vi "MathCad_Easy_NumComplex_Get_Var.vi"(8 "error in (no error)":errorcluster, 9 "Variable  Name":string, 11 "Mathcad Reference":T1) -> (0 "error out":errorcluster, 1 "value":cdb format="%.2f", 3 "Mathcad Reference":T1)   [LabVIEW 2015]
doc: "Sets a Numeric value in Mathcad. You can also use this VI to reset a variable that has already been set once. It is only dependent upon the variable name. The variable won't appear in the Mathcad worksheet, but is defined at the very beginning of the worksheet.\nInputs \n Wrksht Ref--ActiveX Reference to Mathcad Worksheet Class\n Data In--Name and Value of Variable to Set\n Cluster (2 elements)\n Value (Double)\n New Variable Name(String)\nOutputs \n Wrksht Ref--ActiveX Reference to Mathcad Worksheet Class"
uses:
  Mathcad Reference.ctl
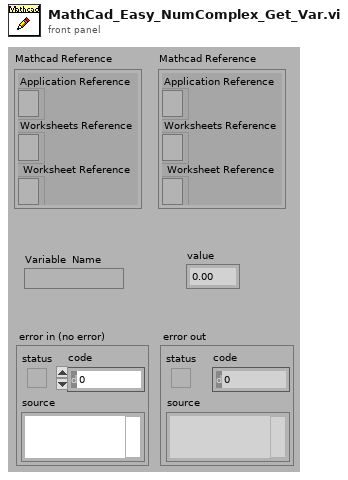
[diagram p1: front panel]
types:
  T1 = typedef "Mathcad Reference.ctl" = cluster{"Application Reference":refnum<k7>, "Worksheets Reference":refnum<k7>, " Worksheet Reference":refnum<k7>}
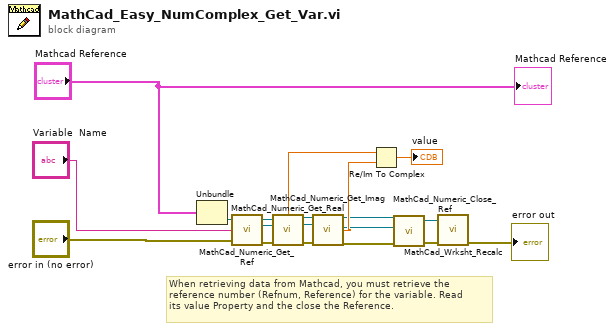
[diagram p0: block diagram]
diagram:
  # "When retrieving data from Mathcad, you must retrieve the \nreference number (Refnum, Reference) for the variable. Read \nits value Property and the close the Reference."
  n1 = Unbundle("Mathcad Reference") -> ("Worksheet Reference"=w11:refnum<k7>)  [unwired: 2 out]
  n2 = call "MathCad_Numeric_Get_Ref.vi"("error in (no error)"="error in (no error)", "Variable  Name"="Variable  Name", "Worksheet Reference In"=w11) -> ("error out"=w16:errorcluster, "Mathcad.INumericValue Refnum"=w17:refnum<k7>, "Worksheet Reference Out"=w18:refnum<k7>)
  n3 = call "MathCad_Numeric_Get_Real.vi"("Worksheet Reference In"=w18, "Mathcad.INumericValue Refnum In"=w17, "error in"=w16) -> ("value"=w7:dbl, "Worksheet Reference Out"=w9:refnum<k7>, "Mathcad.INumericValue Refnum Out"=w8:refnum<k7>, "error out"=w10:errorcluster)  [unwired: 9 in]
  n4 = call "MathCad_Numeric_Get_Imag.vi"("Worksheet Reference In"=w9, "Mathcad.INumericValue Refnum In"=w8, "error in"=w10) -> ("Worksheet Reference Out"=w4:refnum<k7>, "Mathcad.INumericValue Refnum Out"=w3:refnum<k7>, "Imag"=w6:dbl, "error out"=w2:errorcluster)  [unwired: 9 in]
  n5 = Re/Im To Complex(1:w6, 2:w7) -> (0:→"value":cdb)
  n6 = call "MathCad_Numeric_Close_Ref.vi"("error in"=w2, "Mathcad.INumericValue Reference"=w3, "IMathcadWorksheet Reference"=w4) -> ("error out"=w15:errorcluster, "IMathcadWorksheet Reference"=w14:refnum<k7>)  [unwired: 2 in]
  n7 = call "MathCad_Wrksht_Recalc.vi"("error in (no error)"=w15, "Worksheet Reference"=w14) -> ("error out"=→"error out":errorcluster)  [unwired: 8 in, 1 out]
  "Mathcad Reference" <- "Mathcad Reference"
